vi "Keithley 27XX Advanced Scan.vi"() -> ()   [LabVIEW 2020]
doc: "This example is similar to the Finite Multi-point Read Example in that it returns the measurement data on a specified range of channels. The additional feature is having different configurations on different channels in the same scan."
uses:
  <instrlib>/Keithley 27XX/Public/Data/Read Multiple Direct.vi
  <instrlib>/Keithley 27XX/Keithley 27XX.lvlib
panel:
  in  "Serial Configuration":T1={"Baud Rate (9600)"=9600, "Flow Control (1: XON/XOFF)"=1, "Termination Char (0:CR)"=0} {"Termination Char (0:CR)" items=["CR", "LF", "CRLF (Do not use)", "LFCR (Do not use)"]; "Flow Control (1: XON/XOFF)" items=["None", "XON/XOFF", "RTS/CTS (2701 Only)", "XON/XOFF & RTS/CTS (2701 Only)"]; "Baud Rate (9600)" items=["300"=300, "600"=600, "1200"=1200, "2400"=2400, "4800"=4800, "9600"=9600, "19.2k"=19200, "38.4k (2701 Only)"=38400, "57.6k (2701 Only)"=57600, "115.2k (2701 Only)"=115200]}
  in  "Timeout (30000 milliseconds)":u32=30000
  in  "Scan List B (106:110)":string="106:110"
  in  "Function B (6: Temperature)":u16(ring)=6 items=["DC Voltage", "AC Voltage", "DC Current", "AC Current", "Resistance", "Four-Wire Resistance", "Temperature", "Frequency", "Period", "Continuity"]
  in  "Sample Count (100)":i32=100
  out "Measurement Data":dbl[](array[numeric])
  in  "Function A (0: DC Voltage)":u16(ring) items=["DC Voltage", "AC Voltage", "DC Current", "AC Current", "Resistance", "Four-Wire Resistance", "Temperature (C)", "Frequency", "Period", "Continuity"]
  in  "Scan List A (101:105)":string="101:105"
  in  "VISA resource name":refnum<visa-resource-name>
  # "© 2005 National Instruments Corporation.  ALL RIGHTS RESERVED."
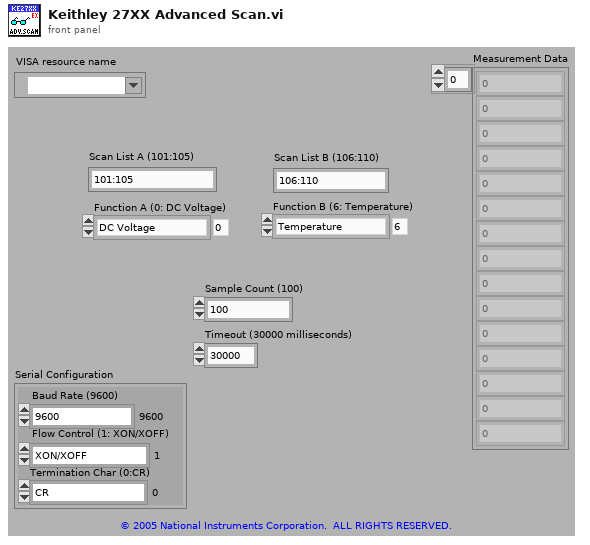
[diagram p1: front panel]
types:
  T1 = cluster{"Baud Rate (9600)":u32, "Flow Control (1: XON/XOFF)":u16, "Termination Char (0:CR)":u16}
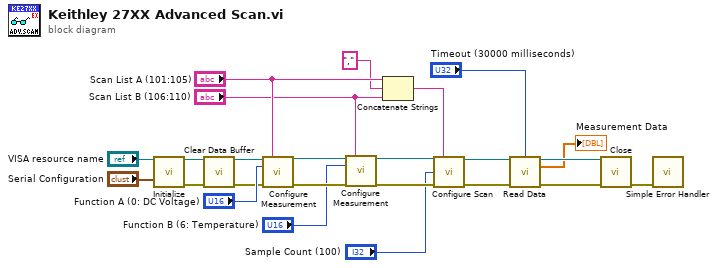
[diagram p0: block diagram]
diagram:
  n1 = call <instrlib>:"Initialize.vi"("VISA resource name"="VISA resource name", "Serial Configuration"="Serial Configuration") -> ("VISA resource name out"=w16:refnum<visa-resource-name>, "error out"=w17:errorcluster)  [unwired: 12 in]
  n2 = call <instrlib>:"Clear Data Buffer.vi"("VISA resource name"=w16, "error in (no error)"=w17) -> ("VISA resource name out"=w19:refnum<visa-resource-name>, "error out"=w18:errorcluster)  [unwired: 12 in]
  n3 = call <instrlib>:"Configure Measurement.vi"("VISA resource name"=w19, "Scan List (Empty)"="Scan List A (101:105)", "Function (0: DC Voltage)"="Function A (0: DC Voltage)", "error in (no error)"=w18) -> ("VISA resource name out"=w12:refnum<visa-resource-name>, "error out"=w13:errorcluster)  [unwired: 10 in]
  n4 = call <instrlib>:"Configure Measurement.vi"("VISA resource name"=w12, "Scan List (Empty)"="Scan List B (106:110)", "Function (0: DC Voltage)"="Function B (6: Temperature)", "error in (no error)"=w13) -> ("VISA resource name out"=w11:refnum<visa-resource-name>, "error out"=w10:errorcluster)  [unwired: 10 in]
  n5 = Concatenate Strings("Scan List A (101:105)", "," ("string"), "Scan List B (106:110)") -> (w6:string)
  n6 = call <instrlib>:"Configure Scan.vi"("VISA resource name"=w11, "Channel List (101:110)"=w6, "Sample Count (100)"="Sample Count (100)", "error in (no error)"=w10) -> ("VISA resource name out"=w14:refnum<visa-resource-name>, "error out"=w15:errorcluster)  [unwired: 10 in]
  n7 = call-poly <instrlib>:"Read Data.vi"("VISA resource name"=w14, "Timeout (30000 milliseconds)"="Timeout (30000 milliseconds)", "error in (no error)"=w15) -> ("VISA resource name out"=w22:refnum<visa-resource-name>, "Measurement Data"=→"Measurement Data":dbl[], "error out"=w21:errorcluster)  [unwired: 7 in, 3 out]
  n8 = call <instrlib>:"Close.vi"("VISA resource name"=w22, "error in (no error)"=w21) -> ("error out"=w20:errorcluster)  [unwired: 13 in]
  n9 = call <vilib>:"Simple Error Handler.vi"("error in (no error)"=w20) -> ()  [unwired: 4 in, 5 out]
